vi "IT6700H Run List.vi"() -> ()   [LabVIEW 2015]
uses:
  <instrlib>/IT6700H/IT6700H.lvlib
panel:
  in  "List Step Count":i32=3 min=1
  in  "Loop count":i32=1 min=0
  in  "List Timer":i32=3 min=0
  in  "Trigger Current Limit (1.0 A)":dbl=1.0 format="%.2g"
  in  "Trigger Voltage Limit (1.0 V)":dbl=1.0 format="%.2g"
  in  "Serial Configuration":T1={"Baud Rate"=9600, "Parity"=0, "Data Bits"=8, "Stop Bits"=10, "Flow Control"=0} {"Flow Control" items=["None", "XON/XOFF", "RTS/CTS", "XON/XOFF & RTS/CTS", "DTR/DSR", "XON/XOFF & DTR/DSR"]; "Stop Bits" items=["1.0"=10, "1.5"=15, "2.0"=20]; "Data Bits" items=["7"=7, "8"=8]; "Parity" items=["None", "Odd", "Even", "Mark", "Space"]; "Baud Rate" items=["300"=300, "600"=600, "1200"=1200, "2400"=2400, "4800"=4800, "9600"=9600, "19200"=19200]}
  in  "VISA resource name":refnum<visa-resource-name>
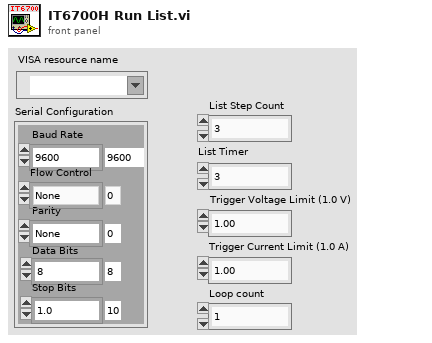
[diagram p1: front panel]
types:
  T1 = cluster{"Baud Rate":u32, "Parity":u16, "Data Bits":u16, "Stop Bits":u16, "Flow Control":u16}
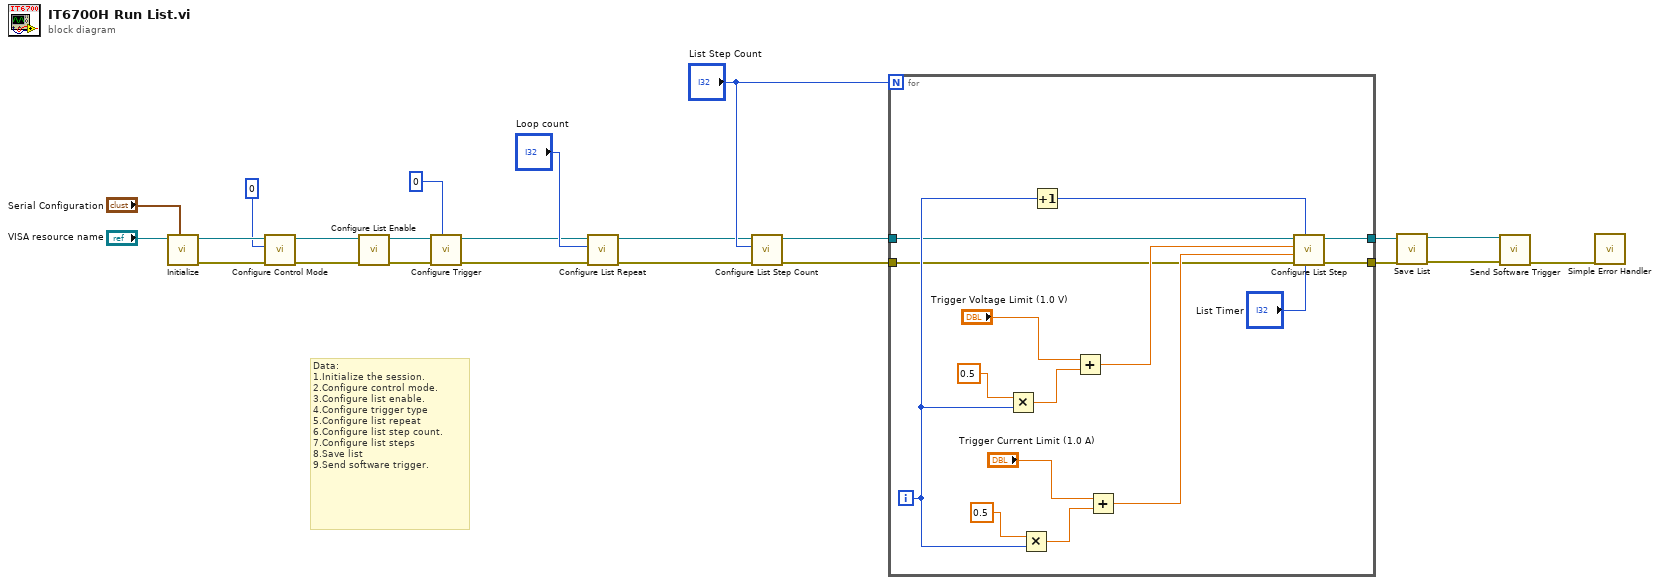
[diagram p0: block diagram]
diagram:
  # "Data:\n1.Initialize the session.\n2.Configure control mode.\n3.Configure list enable.\n4.Configure trigger type\n5.Configure list repeat\n6.Configure list step count.\n7.Configure list steps\n8.Save list\n9.Send software trigger."
  n1 = call <instrlib>:"Initialize.vi"("Serial Configuration"="Serial Configuration", "VISA resource name"="VISA resource name") -> ("error out"=w4:errorcluster, "VISA resource name out"=w5:refnum<visa-resource-name>)  [unwired: 8 in]
  n2 = call <instrlib>:"Configure Control Mode.vi"("error in (no error)"=w4, "Mode  (0: Remote)"=0, "VISA resource name"=w5) -> ("error out"=w2:errorcluster, "VISA resource name out"=w3:refnum<visa-resource-name>)  [unwired: 7 in]
  n3 = call <instrlib>:"Configure List Enable.vi"("error in (no error)"=w2, "VISA resource name"=w3) -> ("error out"=w16:errorcluster, "VISA resource name out"=w17:refnum<visa-resource-name>)  [unwired: 8 in]
  n4 = call <instrlib>:"Configure Trigger.vi"("Trigger Type(0: Bus)"=0, "error in (no error)"=w16, "VISA resource name"=w17) -> ("error out"=w12:errorcluster, "VISA resource name out"=w13:refnum<visa-resource-name>)  [unwired: 7 in]
  n5 = call <instrlib>:"Configure List Repeat.vi"("error in (no error)"=w12, "Loop count (1)"="Loop count", "VISA resource name"=w13) -> ("error out"=w10:errorcluster, "VISA resource name out"=w11:refnum<visa-resource-name>)  [unwired: 7 in]
  n6 = call <instrlib>:"Configure List Step Count.vi"("error in (no error)"=w10, "List Total"="List Step Count", "VISA resource name"=w11) -> ("error out"=w19:errorcluster, "VISA resource name out"=w20:refnum<visa-resource-name>)  [unwired: 7 in]
  n7 = for {
    N: "List Step Count" -> [_]
    tunnel: w20 -> [w28]
    tunnel: w19 -> [w27]
    tunnel: [w26] -> w8
    tunnel: [w25] -> w9
    i -> [w30]
    n8 = Multiply(x=0.5, y=w30) -> (x*y=w37:dbl)
    n9 = Multiply(x=0.5, y=w30) -> (x*y=w33:dbl)
    n10 = Increment(x=w30) -> (x+1=w29:i32)
    n11 = Add(x="Trigger Voltage Limit (1.0 V)", y=w37) -> (x+y=w35:dbl)
    n12 = Add(x="Trigger Current Limit (1.0 A)", y=w33) -> (x+y=w31:dbl)
    n13 = call <instrlib>:"Configure List Step.vi"("List Timer"="List Timer", "List Index"=w29, "error in (no error)"=w27, "Trigger Current Limit (0.0 A)"=w31, "Trigger Voltage Limit (0.0 V)"=w35, "VISA resource name"=w28) -> ("error out"=w25:errorcluster, "VISA resource name out"=w26:refnum<visa-resource-name>)  [unwired: 4 in]
  }
  n14 = call <instrlib>:"Save List.vi"("error in (no error)"=w9, "VISA resource name"=w8) -> ("error out"=w6:errorcluster, "VISA resource name out"=w7:refnum<visa-resource-name>)  [unwired: 8 in]
  n15 = call <instrlib>:"Send Software Trigger.vi"("error in (no error)"=w6, "VISA resource name"=w7) -> ("error out"=w21:errorcluster)  [unwired: 8 in, 1 out]
  n16 = call <vilib>:"Simple Error Handler.vi"("error in (no error)"=w21) -> ()  [unwired: 4 in, 5 out]
